vi "Show Windows Task List.vi"(8 "error in (no error)":errorcluster) -> (0 "error out":errorcluster)   [LabVIEW 2020, in "Winevent.lvlib"]
doc: "This VI will show the Windows Task List.\n\nIf the Install Keyboard Filter.vi has been used to disable the Task List, this VI will not display the Task List."
uses:
  Winevent.lvlib
  user32.dll
  Win Util New/Win Util New.lvlib
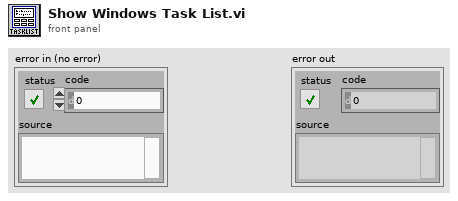
[diagram p1: front panel]
types:
  T1 = enum8{"Maximize Window", "Minimize Window", "Show Task List", "Start Screen Saver", "Quit Application"}
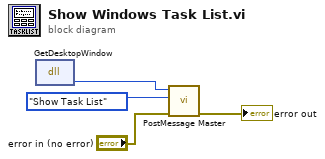
[diagram p0: block diagram]
diagram:
  n1 = dll-call lib="user32.dll" fn="GetDesktopWindow"() -> ("hWndDesktop"=w1:u32)  [unwired: 3 in, 2 out]
  n2 = call "PostMessage Master.vi"("error in"="error in (no error)", "Function"=T1."Show Task List", "window refnum"=w1) -> ("error out"=→"error out":errorcluster)  [unwired: 7 in, 1 out]
